vi "Script Editor Dialog.vi"(5 "VI Refnum":refnum<vi>, 7 "Name (\"\" to Use Uuid)":string="script_editor", 8 "Error In":errorcluster caption="Error in (no error)", 11 "Script":string="Data: Initialize\nInitialize Core Data\nEvents: Register\nUI: Initialize\nUI: Front Panel State >> Open\nstatus@a >> api@b -><register>") -> (0 "Error Out":errorcluster, 3 "Script Out":string)   [LabVIEW 2017]
uses:
  AdvanceAPI/CSM - Keywords.vi
  _Polymophic/CSM - Replace Marks in Messages.vi
  _Shared/Trim Single-line Text.vi
  Communicable State Machine.lvlib
  _ui/csm-ui-support.lvlib
panel:
  in  "Script List":i32(listbox)
  in  "Add Back":bool
  in  "Delete":bool
  in  "Add Front":bool
  in  "Replace":bool
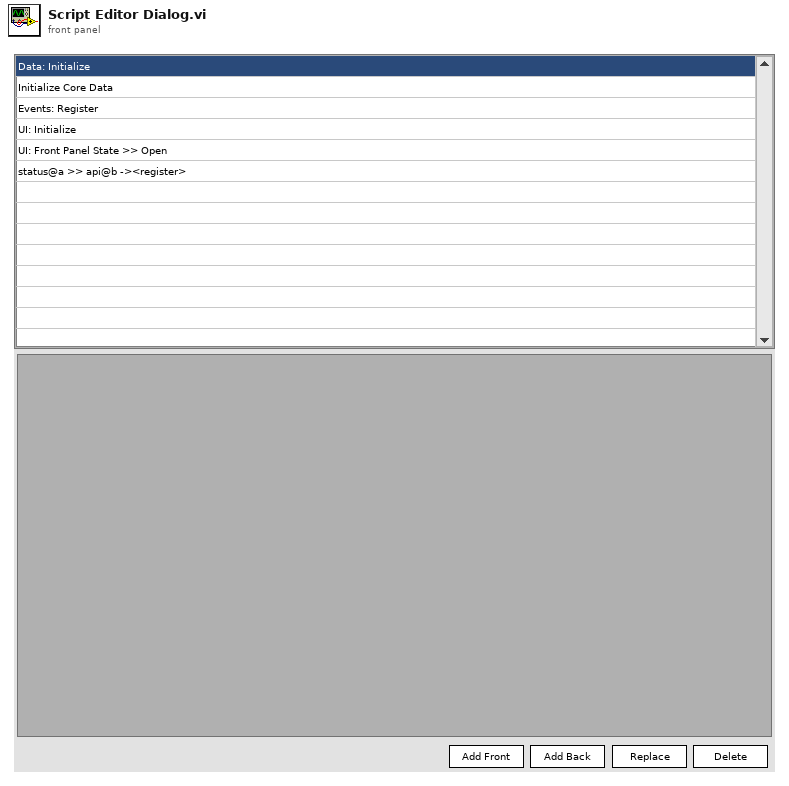
[diagram p1: front panel]
types:
  T1 = enum32{"Invalid", "Standard", "Closed", "Hidden", "Minimized", "Maximized"}
  T2 = enum32{"invalid app kind", "Development System", "Run Time System", "Student Edition", "Embedded LabVIEW", "Evaluation", "Custom"}
  T3 = typedef "Communicable State Machine.lvlib/_CSM_Response Source Message.ctl" = cluster{"‘State":string, "’Arguments":string, "’Error":errorcluster}
  T4 = cluster{"Current VI Reference":refnum<vi>, "Close Panel on Exit?":bool}
  T5 = cluster{"Core":cluster{"Current VI Reference":refnum<vi>, "Close Panel on Exit?":bool}, "Script":string}
  T6 = typedef "LVRectTypeDef.ctl" = cluster{"Left":i16, "Top":i16, "Right":i16, "Bottom":i16}
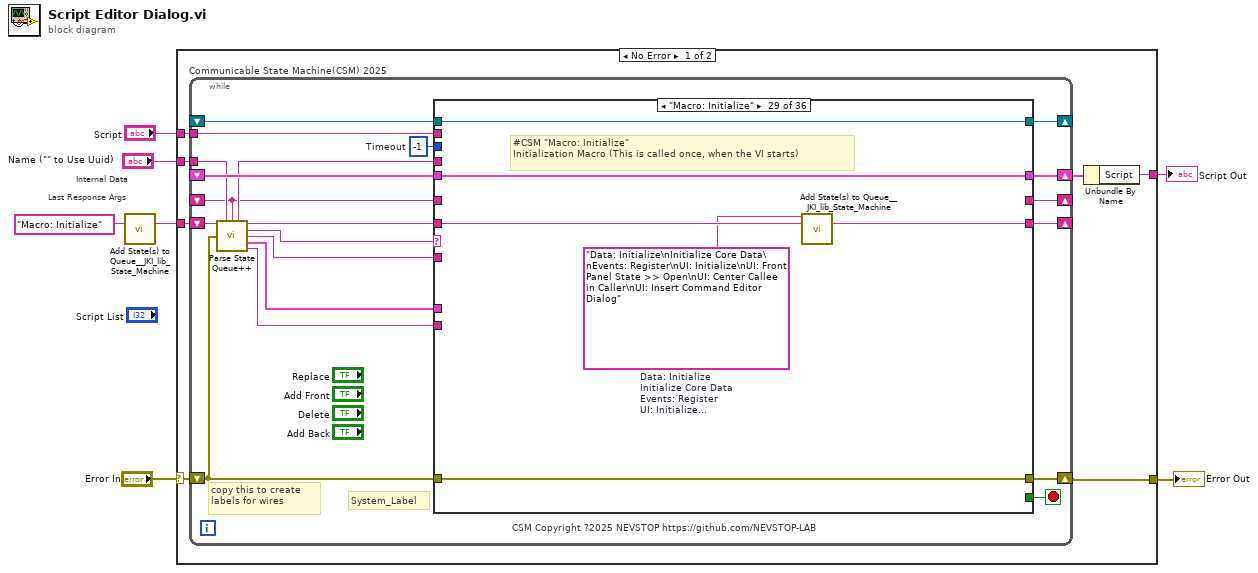
[diagram p0: block diagram]
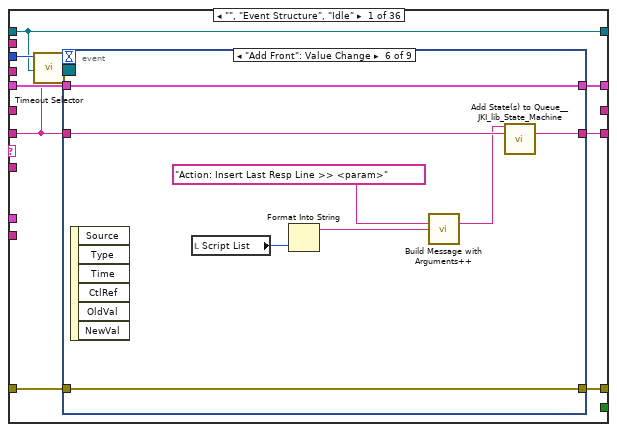
[diagram p2: hidden frame]
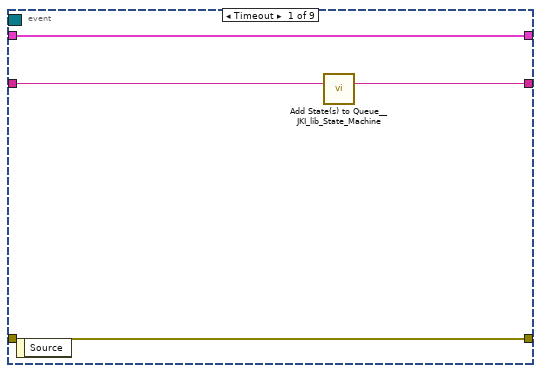
[diagram p3: hidden frame]
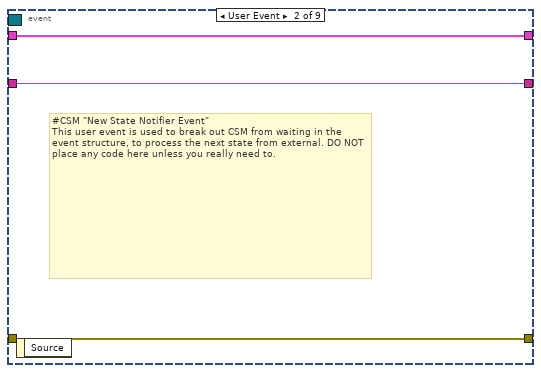
[diagram p4: hidden frame]
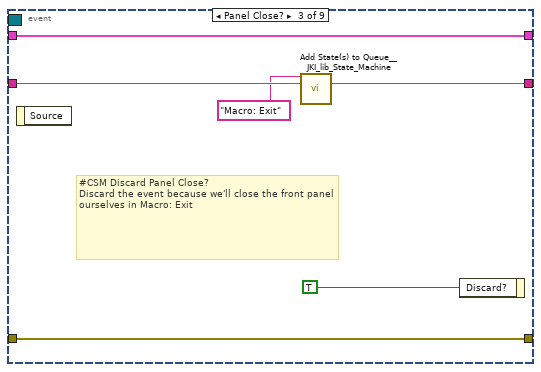
[diagram p5: hidden frame]
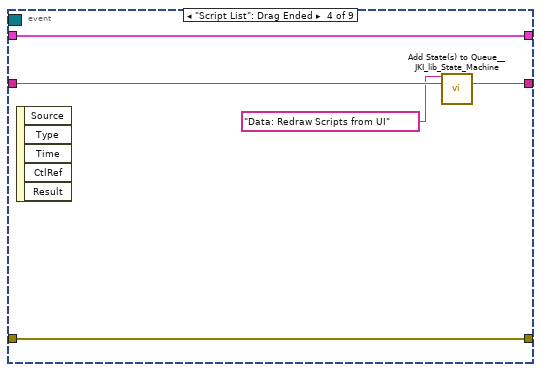
[diagram p6: hidden frame]
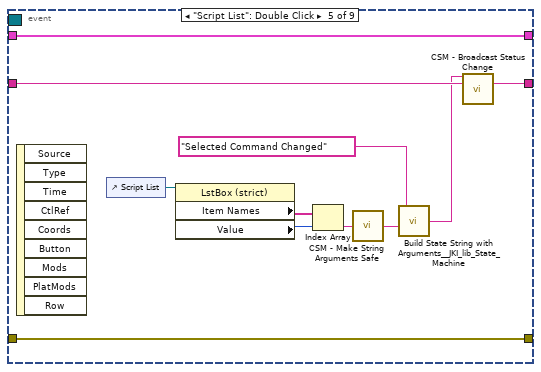
[diagram p7: hidden frame]
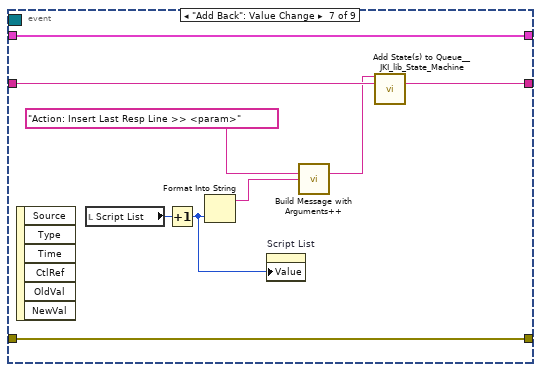
[diagram p8: hidden frame]
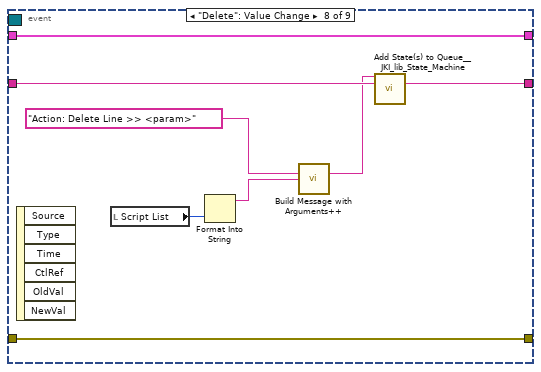
[diagram p9: hidden frame]
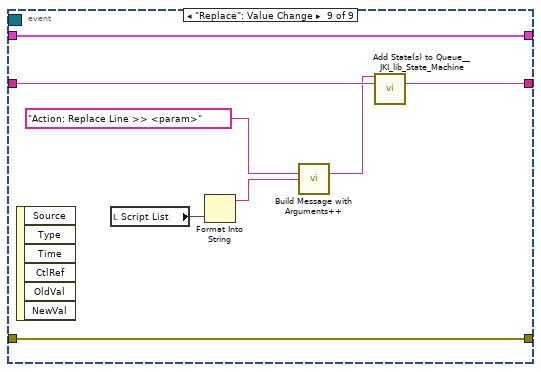
[diagram p10: hidden frame]
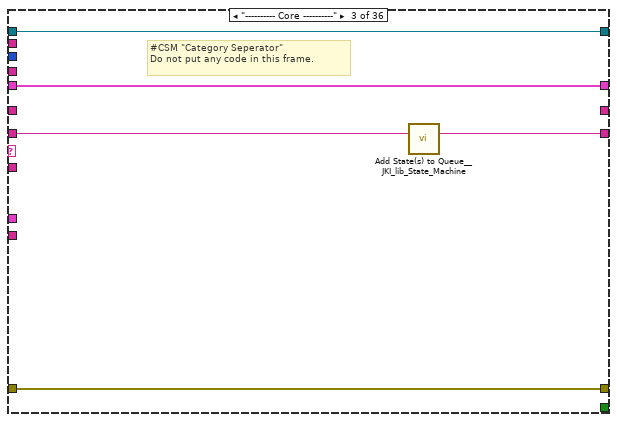
[diagram p12: hidden frame]
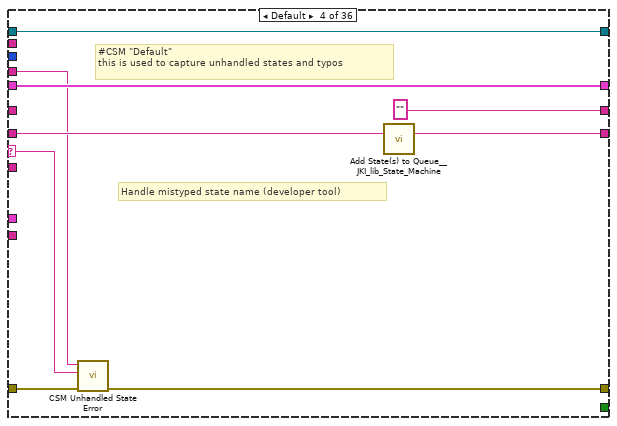
[diagram p13: hidden frame]
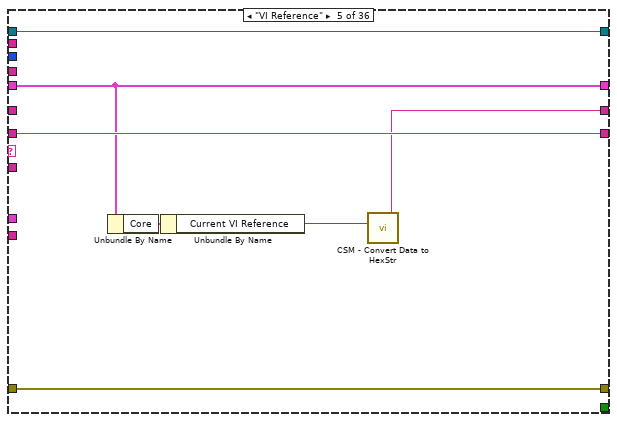
[diagram p14: hidden frame]
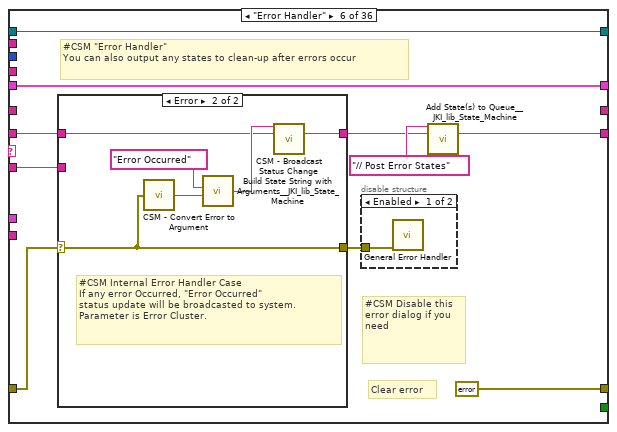
[diagram p15: hidden frame]
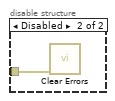
[diagram p16: hidden frame]
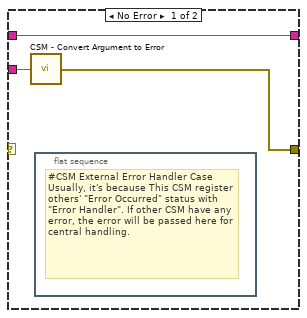
[diagram p17: hidden frame]
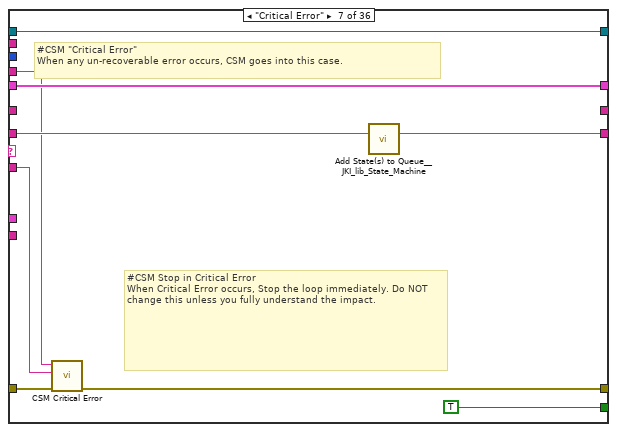
[diagram p18: hidden frame]
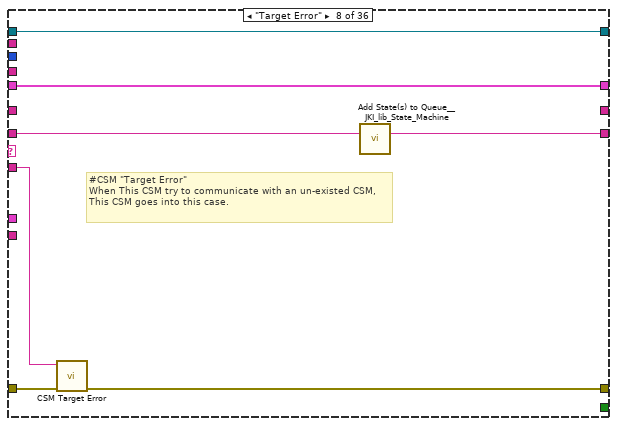
[diagram p19: hidden frame]
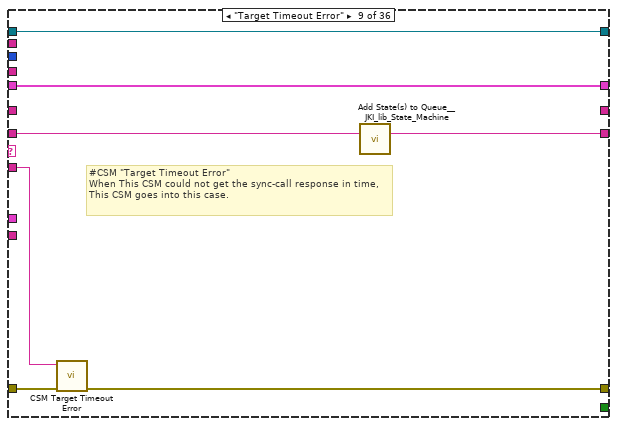
[diagram p20: hidden frame]
diagram:
  # "Last Response Args"
  # "Internal Data"
  n1 = call <vilib>:"Add State(s) to Queue__JKI_lib_State_Machine.vi"("State(s) in (\"\")"="Macro: Initialize" ("Init State(\"Macro: Initialize\")")) -> ("States Out"=w7:string)  [unwired: 14 in]
  n2 = case shown="No Error" "Error In" {
    selector: "Error In" -> [w11 w492]
    tunnel: w7 -> [w14 _]
    tunnel: "Name (\"\" to Use Uuid)" -> [w13 _]
    tunnel: [w12 w492] -> w4
    tunnel: [w9 w491] -> w2
    tunnel: "Script" -> [w8 w491]
    frame No Error {
      n3 = while "Communicable State Machine(CSM) 2025" {
        shift-right: [w29] -> w10
        shift-left: _ -> [w28]
        shift-right: [w32] -> w12
        shift-left: w11 -> [w26]
        shift-right: [w31] -> _
        shift-left: w14 -> [w33]
        tunnel: w13 -> [w22]
        shift-right: [w25] -> _
        shift-left: _ -> [w16]
        shift-right: [w24] -> _
        shift-left: _ -> [w23]
        tunnel: w8 -> [w15]
        stop <- w30 stop-if-true
        w27 = -1  # Timeout
        # "copy this to create labels for wires"
        # "System_Label"
        # "CSM Copyright ?2025 NEVSTOP https://github.com/NEVSTOP-LAB"
        n4 = call "Parse State Queue++.vi"("State Queue"=w33, "Name (\"\" to Use UUID)"=w22, "Response Arguments"=w16, "Previous Error"=w26) -> ("Name Used"=w17:string, "Remaining States"=w34:string, "Current State"=w21:string, "Arguments"=w20:string, "Additional Information"=w19:T3, "Source CSM"=w18:string)  [unwired: 6 in]
        n5 = case shown="\"Macro: Initialize\"" w21 {
          selector: w21 -> [_ _ _ w117 _ _ _ _ _ _ _ _ _ _ _ _ _ _ _ _ _ _ _ _ _ _ _ _ _ _ _ _ _ _ _ _]
          tunnel: w34 -> [w35 w108 w114 w122 w129 w135 w158 w164 w171 w180 w193 w208 w214 w219 w226 w233 w241 w246 w253 w257 w263 w270 w278 w281 w293 w309 w382 w404 w410 w424 w427 w430 w442 w460 w478 w490]
          tunnel: w20 -> [_ _ _ _ _ w134 w153 w163 w170 w179 _ _ _ _ _ _ _ _ _ _ _ _ _ _ w288 w303 _ _ _ _ _ w432 _ w456 w473 w485]
          tunnel: w28 -> [w42 w107 w111 w120 w128 w139 w159 w166 w173 w182 w192 w201 w212 w216 _ w232 w236 w243 w252 w256 w260 w266 w276 w285 w291 w305 w399 w401 w407 w421 w426 w436 w439 w458 w475 w487]
          tunnel: [w41 w109 w112 w115 w130 errorcluster {"status"=FALSE, "code"=0, "source"=""} ("error out") w154 w161 w168 w185 w194 w205 w211 w217 w223 w234 w237 w244 w247 w255 w261 w268 w279 w286 w289 w306 w381 w402 w408 w422 w428 w437 w440 w447 w476 w488] -> w32
          tunnel: w26 -> [w40 w109 w112 w123 w130 w136 w160 w162 w169 _ w194 w205 w211 w217 w223 w234 w238 w244 _ w258 w261 w268 w279 w286 w290 w307 _ w402 w408 w422 w428 w437 w440 _ w476 w488]
          tunnel: [w43 w108 w113 w121 w129 w131 w157 w167 w174 w181 w193 w207 w213 w218 w225 w233 w240 w245 w253 w257 w262 w269 w278 w282 w292 w308 w383 w403 w409 w423 w427 w431 w441 w459 w477 w489] -> w31
          tunnel: [_ _ _ _ _ _ TRUE _ _ _ _ _ TRUE _ _ _ _ _ _ _ _ _ _ _ _ _ _ _ _ _ _ _ _ _ _ _] -> w30
          tunnel: [w39 w107 w111 w120 w128 w139 w159 w166 w173 w183 w192 w206 w212 w216 w224 w228 w236 w243 w252 w256 w260 w266 w276 w285 w291 w305 w399 w401 w407 w421 w426 w434 w439 w458 w475 w487] -> w29
          tunnel: w27 -> [w38 _ _ _ _ _ _ _ _ _ _ _ _ _ _ _ _ _ _ _ _ _ _ _ _ _ _ _ _ _ _ _ _ _ _ _]
          tunnel: w18 -> [_ _ _ _ _ _ _ _ _ w177 _ _ _ _ _ _ _ _ _ _ _ _ _ _ _ _ _ _ _ _ _ _ _ _ _ _]
          tunnel: w19 -> [_ _ _ _ _ _ _ _ _ w184 _ _ _ _ _ _ _ _ _ _ _ _ _ _ _ _ _ _ _ _ _ _ _ _ _ _]
          tunnel: [_ _ _ "" w124 _ _ _ _ _ _ _ _ _ _ _ _ _ _ _ _ _ _ _ _ _ _ _ _ _ _ _ _ _ _ _] -> w25
          tunnel: [w37 w106 w110 w118 w127 w138 w155 w165 w172 w186 w191 w195 w209 w215 w221 w231 w235 w242 w251 w254 w259 w267 w277 w284 w287 w302 w398 w400 w405 w414 w425 w435 w438 w457 w474 w486] -> w24
          tunnel: w23 -> [w37 w106 w110 w118 w127 w138 w155 w165 w172 w186 w191 w195 w209 w215 w221 w231 w235 w242 _ w254 w259 w267 w277 w284 w287 w302 w398 w400 w405 w414 w425 w435 w438 w457 w474 w486]
          tunnel: w17 -> [_ _ _ w116 _ _ w152 _ _ _ _ _ _ _ _ _ _ _ w250 _ _ _ _ _ _ _ w387 _ _ w413 _ _ _ w446 w464 _]
          tunnel: w16 -> [_ _ _ _ _ _ _ _ _ _ _ _ _ _ _ _ _ _ _ _ _ _ _ _ _ _ _ _ _ _ _ _ _ _ _ _]
          tunnel: w15 -> [_ _ _ _ _ _ _ _ _ _ _ _ _ _ w220 _ _ _ _ _ _ _ _ _ _ _ _ _ _ _ _ _ _ _ _ _]
          frame "", "Event Structure", "Idle" {
            n6 = call "Timeout Selector.vi"("Remaining States"=w35, "Timeout Expected"=w38) -> ("Timeout"=w36:i32)  [unwired: 5 in]
            n7 = event shown="[5] \"Add Front\": Value Change" {
              selector: w37 -> [_ _ _ _ _ _ _ _ _]
              dyn-events: _ -> [_ _ _ _ _ _ _ _ _]
              timeout: w36 -> [_ _ _ _ _ _ _ _ _]
              tunnel: w35 -> [w47 w49 w56 w58 w69 w77 w86 w94 w102]
              tunnel: [w46 w49 w55 w59 w70 w78 w87 w95 w103] -> w43
              tunnel: w42 -> [w44 w50 w53 w60 w71 w79 w88 w96 w104]
              tunnel: [w45 w48 w54 w61 w72 w80 w89 w97 w105] -> w41
              tunnel: w40 -> [w45 w48 w54 w61 w72 w80 w89 w97 w105]
              tunnel: [w44 w50 w53 w60 w71 w79 w88 w96 w104] -> w39
              event Timeout {
                n8 = event-data() -> ()  [unwired: 1 in, 1 out]
                n9 = call <vilib>:"Add State(s) to Queue__JKI_lib_State_Machine.vi"("State(s) in (\"\")"=w47) -> ("States Out"=w46:string)  [unwired: 14 in]
              }
              event User Event {
                # "#CSM \"New State Notifier Event\"\nThis user event is used to break out CSM from waiting in the event structure, to process the next state from external. DO NOT place any code here unless you really need to."
                n10 = event-data() -> ()  [unwired: 1 in, 1 out]
              }
              event Panel Close? {
                # "#CSM Discard Panel Close?\nDiscard the event because we'll close the front panel ourselves in Macro: Exit"
                n11 = event-data() -> ()  [unwired: 1 in, 1 out]
                n12 = call <vilib>:"Add State(s) to Queue__JKI_lib_State_Machine.vi"("State(s) in Front (\"\")"="Macro: Exit", "State(s) in (\"\")"=w56) -> ("States Out"=w55:string)  [unwired: 13 in]
                n13 = event-data("Discard?"=TRUE) -> ()  [unwired: 1 in, 1 out]
              }
              event "Script List": Drag Ended {
                n14 = event-data() -> ()  [unwired: 1 in, 5 out]
                n15 = call <vilib>:"Add State(s) to Queue__JKI_lib_State_Machine.vi"("State(s) in Front (\"\")"="Data: Redraw Scripts from UI" ("State(s) in Front (\"\")"), "State(s) in (\"\")"=w58) -> ("States Out"=w59:string)  [unwired: 13 in]
              }
              event "Script List": Double Click {
                n16 = event-data() -> ()  [unwired: 1 in, 9 out]
                n17 = control-ref of="Script List"() -> (w65:refnum<vi>)
                n18 = property class="LstBox (strict)"(reference=w65) -> ("Item Names"=w68:string[], "Value"=w67:i32)  [unwired: 1 in, 2 out]
                n19 = Index Array(array=w68, index=w67) -> (element=w66:string)
                n20 = call "CSM - Make String Arguments Safe.vi"("Argument String"=w66) -> ("Safe Argument String"=w64:string)  [unwired: 8 in]
                n21 = call <vilib>:"Build State String with Arguments__JKI_lib_State_Machine.vi"("Arguments (\"\")"=w64, "State"="Selected Command Changed") -> ("State with Arguments"=w62:string)  [unwired: 4 in]
                n22 = call "CSM - Broadcast Status Change.vi"("Status With Arguments"=w62, "State Queue"=w69) -> ("Remaining States"=w70:string)  [unwired: 13 in]
              }
              event "Add Front": Value Change {
                n23 = event-data() -> ()  [unwired: 1 in, 6 out]
                n24 = local read "Script List"() -> (w74:i32)
                n25 = Format Into String(w74) -> (resulting string=w73:string)  [unwired: 3 in, 1 out]
                n26 = call-poly "Build Message with Arguments++.vi"("States With Replace Token"="Action: Insert Last Resp Line >> <param>" ("State(s) in Front (\"\")"), "<param>"=w73) -> ("States"=w75:string)  [unwired: 13 in]
                n27 = call <vilib>:"Add State(s) to Queue__JKI_lib_State_Machine.vi"("State(s) in Front (\"\")"=w75, "State(s) in (\"\")"=w77) -> ("States Out"=w78:string)  [unwired: 13 in]
              }
              event "Add Back": Value Change {
                n28 = event-data() -> ()  [unwired: 1 in, 6 out]
                n29 = local read "Script List"() -> (w83:i32)
                n30 = Increment(x=w83) -> (x+1=w81:i32)
                n31 = Format Into String(w81) -> (resulting string=w82:string)  [unwired: 3 in, 1 out]
                n32 = property on="Script List" class="LstBox (strict)"("Value"=w81) -> ()  [unwired: 2 in, 2 out]
                n33 = call-poly "Build Message with Arguments++.vi"("States With Replace Token"="Action: Insert Last Resp Line >> <param>" ("State(s) in Front (\"\")"), "<param>"=w82) -> ("States"=w84:string)  [unwired: 13 in]
                n34 = call <vilib>:"Add State(s) to Queue__JKI_lib_State_Machine.vi"("State(s) in Front (\"\")"=w84, "State(s) in (\"\")"=w86) -> ("States Out"=w87:string)  [unwired: 13 in]
              }
              event "Delete": Value Change {
                n35 = event-data() -> ()  [unwired: 1 in, 6 out]
                n36 = local read "Script List"() -> (w91:i32)
                n37 = Format Into String(w91) -> (resulting string=w90:string)  [unwired: 3 in, 1 out]
                n38 = call-poly "Build Message with Arguments++.vi"("States With Replace Token"="Action: Delete Line >> <param>" ("State(s) in Front (\"\")"), "<param>"=w90) -> ("States"=w92:string)  [unwired: 13 in]
                n39 = call <vilib>:"Add State(s) to Queue__JKI_lib_State_Machine.vi"("State(s) in Front (\"\")"=w92, "State(s) in (\"\")"=w94) -> ("States Out"=w95:string)  [unwired: 13 in]
              }
              event "Replace": Value Change {
                n40 = event-data() -> ()  [unwired: 1 in, 6 out]
                n41 = local read "Script List"() -> (w99:i32)
                n42 = Format Into String(w99) -> (resulting string=w98:string)  [unwired: 3 in, 1 out]
                n43 = call-poly "Build Message with Arguments++.vi"("States With Replace Token"="Action: Replace Line >> <param>" ("State(s) in Front (\"\")"), "<param>"=w98) -> ("States"=w100:string)  [unwired: 13 in]
                n44 = call <vilib>:"Add State(s) to Queue__JKI_lib_State_Machine.vi"("State(s) in Front (\"\")"=w100, "State(s) in (\"\")"=w102) -> ("States Out"=w103:string)  [unwired: 13 in]
              }
            }
          }
          frame "CSM Documentation" {
            # "#CSM README FIRST\n\nCommunicable State Machine(CSM) is a LabVIEW application framework that builds upon JKI State Machine(JKISM). It follows the pattern of JKISM and extends the keywords to describe message communication between modules, including concepts such as Sync-Message, Async-Message, Subscription/Unsubscription of status - essential elements for creating reusable code modules. For more information, please visit the CSM wiki: https://nevstop-lab.github.io/CSM-Wiki/\n\nFor instructions on JKI State Machine, visit: http://jki.net/state-machine/\nFor information about CSM, visit: https://github.com/NEVSTOP-LAB"
            # "#CSM \"Documentation\"\nCase for holding CSM Documenation"
          }
          frame "---------- Core ----------" {
            # "#CSM \"Category Seperator\"\nDo not put any code in this frame."
            n45 = call <vilib>:"Add State(s) to Queue__JKI_lib_State_Machine.vi"("State(s) in (\"\")"=w114) -> ("States Out"=w113:string)  [unwired: 14 in]
          }
          frame Default {
            # "#CSM \"Default\"\nthis is used to capture unhandled states and typos"
            # "Handle mistyped state name (developer tool)"
            n46 = call "CSM Unhandled State Error.vi"("error in (no error)"=w123, "Undefined State"=w117, "CSM Name"=w116) -> ("error out"=w115:errorcluster)  [unwired: 8 in]
            n47 = call <vilib>:"Add State(s) to Queue__JKI_lib_State_Machine.vi"("State(s) in (\"\")"=w122) -> ("States Out"=w121:string)  [unwired: 14 in]
          }
          frame "VI Reference" {
            n48 = Unbundle By Name(w128) -> ("Core"=w126:T4)
            n49 = Unbundle By Name(w126) -> ("Current VI Reference"=w125:refnum<vi>)
            n50 = call "CSM - Convert Data to HexStr.vi"("Variant"=w125) -> ("HEX String (0-9,A-F)"=w124:string)  [unwired: 8 in]
          }
          frame "Error Handler" {
            # "#CSM Disable this error dialog if you need"
            # "#CSM \"Error Handler\"\nYou can also output any states to clean-up after errors occur"
            # "Clear error"
            n51 = case shown="Error" w136 {
              selector: w136 -> [_ w146]
              tunnel: [w145 w148] -> w132
              tunnel: w135 -> [w145 w147]
              tunnel: w134 -> [w144 _]
              tunnel: [w143 w146] -> w137
              frame No Error {
                n52 = call "CSM - Convert Argument to Error.vi"("Argument"=w144) -> ("Error"=w143:errorcluster)  [unwired: 4 in]
                n53 = flat-sequence {
                  frame #0 {
                    # "#CSM External Error Handler Case\nUsually, it's because This CSM register others' \"Error Occurred\" status with \"Error Handler\". If other CSM have any error, the error will be passed here for central handling."
                  }
                }
              }
              frame Error {
                # "#CSM Internal Error Handler Case \nIf any error Occurred, \"Error Occurred\" \nstatus update will be broadcasted to system.\nParameter is Error Cluster."
                n54 = call "CSM - Convert Error to Argument.vi"("Error"=w146) -> ("Argument"=w150:string)  [unwired: 4 in]
                n55 = call <vilib>:"Build State String with Arguments__JKI_lib_State_Machine.vi"("Arguments (\"\")"=w150, "State"="Error Occurred" ("Status with Arguments")) -> ("State with Arguments"=w149:string)  [unwired: 4 in]
                n56 = call "CSM - Broadcast Status Change.vi"("Status With Arguments"=w149, "State Queue"=w147) -> ("Remaining States"=w148:string)  [unwired: 13 in]
              }
            }
            n57 = disable-structure shown="Enabled" {
              disable-tunnel: w137 -> [w141 w142]
              frame Enabled {
                n58 = call <vilib>:"General Error Handler.vi"("error in (no error)"=w141) -> ()  [unwired: 10 in, 5 out]
              }
              frame Disabled {
                n59 = call <vilib>:"Clear Errors.vi"("error in (no error)"=w142) -> ()  [unwired: 5 in, 2 out]
              }
            }
            n60 = call <vilib>:"Add State(s) to Queue__JKI_lib_State_Machine.vi"("State(s) in Front (\"\")"="// Post Error States", "State(s) in (\"\")"=w132) -> ("States Out"=w131:string)  [unwired: 13 in]
          }
          frame "Critical Error" {
            # "#CSM Stop in Critical Error\nWhen Critical Error occurs, Stop the loop immediately. Do NOT change this unless you fully understand the impact."
            # "#CSM \"Critical Error\"\nWhen any un-recoverable error occurs, CSM goes into this case."
            n61 = call "CSM Critical Error.vi"("error in (no error)"=w160, "Arugments (As Reason)"=w153, "CSM Name"=w152) -> ("error out"=w154:errorcluster)  [unwired: 8 in]
            n62 = call <vilib>:"Add State(s) to Queue__JKI_lib_State_Machine.vi"("State(s) in (\"\")"=w158) -> ("States Out"=w157:string)  [unwired: 14 in]
          }
          frame "Target Error" {
            # "#CSM \"Target Error\"\nWhen This CSM try to communicate with an un-existed CSM, This CSM goes into this case."
            n63 = call "CSM Target Error.vi"("error in (no error)"=w162, "Arguments (As CSM Name)"=w163) -> ("error out"=w161:errorcluster)  [unwired: 9 in]
            n64 = call <vilib>:"Add State(s) to Queue__JKI_lib_State_Machine.vi"("State(s) in (\"\")"=w164) -> ("States Out"=w167:string)  [unwired: 14 in]
          }
          frame "Target Timeout Error" {
            # "#CSM \"Target Timeout Error\"\nWhen This CSM could not get the sync-call response in time, This CSM goes into this case."
            n65 = call "CSM Target Timeout Error.vi"("error in (no error)"=w169, "Arguments (As CSM Name)"=w170) -> ("error out"=w168:errorcluster)  [unwired: 9 in]
            n66 = call <vilib>:"Add State(s) to Queue__JKI_lib_State_Machine.vi"("State(s) in (\"\")"=w171) -> ("States Out"=w174:string)  [unwired: 14 in]
          }
          frame "Async Response", "Response" {
            n67 = Unbundle(w184) -> ("‘State"=w178:string, "’Arguments"=w176:string, "’Error"=w175:errorcluster)
            n68 = case shown="Default" w178 {
              tunnel: [w190] -> w185
              tunnel: w175 -> [w190]
              tunnel: [w189] -> w183
              tunnel: w182 -> [w189]
              tunnel: [w187] -> w181
              tunnel: w180 -> [w188]
              tunnel: w179 -> [_]
              tunnel: w177 -> [_]
              tunnel: w176 -> [_]
              frame Default {
                # "#CSM Response Comments\nAfter Message is executed, CSM goes to this state for receive the response.\n    For Async Message(->), \"Async Response\" is used. This CSM will goes to \"Async Message Posted\" immediately and receive the \"Async Response\" after the callee finishes the message.\n    For Sync Message(@),  This CSM will wait until the message is done and immediately goes to \"Response\""
                # "#CSM \"Async Response\"\nHandle Async-call Response (\"Async Response\" for ->)"
                # "#CSM \"Response\"\nHandle Sync-call Response (\"Response\" for -@)"
                n69 = call <vilib>:"Add State(s) to Queue__JKI_lib_State_Machine.vi"("State(s) in (\"\")"=w188) -> ("States Out"=w187:string)  [unwired: 14 in]
              }
            }
          }
          frame "Async Message Posted" {
            # "#CSM \"Async Message Posted\"\nAfter Async Message is posted (-> or ->| ), CSM goes to this state for post-action.\nYou can use Argument - State to tell which Async Message is called."
          }
          frame "Initialize Core Data" {
            # "#CSM \"Initialize Core Data\"\nThis is used to determine panel behavior on exit"
            # "originally closed?"
            # "exe?"
            # "If panel starts closed or is an EXE, then close it when we exit"
            n70 = property class="VI"() -> ("FP.State"=w198:T1)  [unwired: 2 in, 2 out]
            n71 = property class="App"() -> ("App.Kind"=w204:T2)  [unwired: 2 in, 2 out]
            n72 = control-ref of="Current VI Reference"() -> (w199:refnum<vi>)
            n73 = Equal?(x=w198, y=T1."Closed" ("Front Panel Window:State")) -> (x = y?=w196:bool)
            n74 = Equal?(x=w204, y=T2."Run Time System" ("Application:Kind")) -> (x = y?=w202:bool)
            n75 = Or(x=w196, y=w202) -> (x .or. y?=w200:bool)
            n76 = Bundle By Name(cluster=w201, "Core.Current VI Reference"=w199, "Core.Close Panel on Exit?"=w200) -> (w206:T5)
            n77 = call <vilib>:"Add State(s) to Queue__JKI_lib_State_Machine.vi"("State(s) in (\"\")"=w208) -> ("States Out"=w207:string)  [unwired: 14 in]
          }
          frame "Exit" {
            # "#CSM \"Exit\"\nCase for exiting the loop. No errors that occur here will be handled."
            n78 = call <vilib>:"Add State(s) to Queue__JKI_lib_State_Machine.vi"("State(s) in (\"\")"=w214) -> ("States Out"=w213:string)  [unwired: 14 in]
          }
          frame "---------- Data ----------" {
            # "#CSM \"Category Seperator\"\nDo not put any code in this frame."
            n79 = call <vilib>:"Add State(s) to Queue__JKI_lib_State_Machine.vi"("State(s) in (\"\")"=w219) -> ("States Out"=w218:string)  [unwired: 14 in]
          }
          frame "Data: Initialize" {
            w222 = T4 {"Current VI Reference"=refnum, "Close Panel on Exit?"=FALSE}  # Core
            n80 = Bundle("Core"=w222, "Script"=w220) -> (w224:T5)  [unwired: 1 in]
            n81 = call <vilib>:"Add State(s) to Queue__JKI_lib_State_Machine.vi"("State(s) in (\"\")"=w226) -> ("States Out"=w225:string)  [unwired: 14 in]
          }
          frame "Data: Redraw Scripts from UI" {
            n82 = control-ref of="Script List"() -> (w230:refnum<vi>)
            n83 = property class="LstBox (strict)"(reference=w230) -> ("Item Names"=w229:string[])  [unwired: 1 in, 2 out]
            n84 = call "CSM - Compact Multiple States.vi"("Multiple States"=w229) -> ("States"=w227:string)  [unwired: 9 in]
            n85 = Bundle By Name(cluster=w232, "Script"=w227) -> (w228:T5)
          }
          frame "Data: Cleanup" {
            # "Cleanup any data and references, here.\n(this is called automatically, by the Macro: Exit)"
            n86 = Unbundle By Name(w236) -> ("Core.Current VI Reference"=w239:refnum<vi>)
            n87 = Close Reference(reference=w239, error in (no error)=w238) -> (error out=w237:errorcluster)
            n88 = call <vilib>:"Add State(s) to Queue__JKI_lib_State_Machine.vi"("State(s) in (\"\")"=w241) -> ("States Out"=w240:string)  [unwired: 14 in]
          }
          frame "---------- Events ----------" {
            # "#CSM \"Category Seperator\"\nDo not put any code in this frame."
            n89 = call <vilib>:"Add State(s) to Queue__JKI_lib_State_Machine.vi"("State(s) in (\"\")"=w246) -> ("States Out"=w245:string)  [unwired: 14 in]
          }
          frame "Events: Register" {
            # "#CSM \"Events: Register\"\nRegister user event. New Message Event is registered to break CSM waiting in event structure by default."
            # "#CSM Register New Message Event\nRegister message event to break Waiting in Event structure."
            n90 = call "CSM - Get New State Notifier Event.vi"("Name (\"\" to Use UUID)"=w250) -> ("error out"=w248:errorcluster, "New State Notifier Event"=w249:refnum<user-event>)  [unwired: 9 in]
            n91 = register-events(error in=w248, w249) -> (reference out=w251:refnum<event-registration>, error out=w247:errorcluster)  [unwired: 1 in]
          }
          frame "Events: Unregister" {
            # "#CSM \"Events: Unregister\"\nUnregister user event."
            n92 = Unregister For Events(event registration refnum=w254, error in=w258) -> (error out=w255:errorcluster)
          }
          frame "---------- UI ----------" {
            # "#CSM \"Category Seperator\"\nDo not put any code in this frame."
            n93 = call <vilib>:"Add State(s) to Queue__JKI_lib_State_Machine.vi"("State(s) in (\"\")"=w263) -> ("States Out"=w262:string)  [unwired: 14 in]
          }
          frame "UI: Initialize" {
            # "#CSM \"UI: Initialize\"\nInitialize the User Interface, here.\n(this is called automatically, by the Macro: Init)"
            n94 = Unbundle By Name(w266) -> ("Script"=w265:string)
            n95 = call "CSM - Break Down Multiple States String.vi"("States"=w265) -> ("Multiple States"=w264:string[])  [unwired: 10 in]
            n96 = property on="Script List" class="LstBox (strict)"("Item Names"=w264) -> ()  [unwired: 2 in, 2 out]
            n97 = call <vilib>:"Add State(s) to Queue__JKI_lib_State_Machine.vi"("State(s) in (\"\")"=w270) -> ("States Out"=w269:string)  [unwired: 14 in]
          }
          frame "UI: Center Callee in Caller" {
            n98 = Unbundle By Name(w276) -> ("Core.Current VI Reference"=w273:refnum<vi>)
            n99 = property class="VI"(reference="VI Refnum") -> (error out=w271:errorcluster, "BDWin.Bounds"=w272:T6)  [unwired: 1 in, 1 out]
            n100 = call "Center Callee in Window Bounds.vi"("Callee VI Refnum (Caller)"=w273, "Block Diagram Window:Window Bounds"=w272) -> ("Error Out"=w275:errorcluster)  [unwired: 9 in]
            n101 = call <vilib>:"Clear Errors.vi"("error in (no error)"=w271) -> ()  [unwired: 5 in, 2 out]
            n102 = call <vilib>:"Clear Errors.vi"("error in (no error)"=w275) -> ()  [unwired: 5 in, 2 out]
          }
          frame "UI: Refresh Inputs" {
            n103 = call <vilib>:"Build State String with Arguments__JKI_lib_State_Machine.vi"("State"="") -> ("State with Arguments"=w280:string)  [unwired: 5 in]
            n104 = call <vilib>:"Add State(s) to Queue__JKI_lib_State_Machine.vi"("State(s) in Front (\"\")"=w280, "State(s) in (\"\")"=w281) -> ("States Out"=w282:string)  [unwired: 13 in]
          }
          frame "UI: Cursor Set" {
            # "#CSM \"UI: Cursor Set\"\nSet and Unset Cursor Busy.\n(Usage: \"UI: Cursor Set >> Busy|Idle\")"
            # "Argument"
            n105 = disable-structure shown="Default" {
              disable-tunnel: w290 -> [w296 w301]
              disable-tunnel: [w295 w301] -> w289
              disable-tunnel: w288 -> [w294 _]
              frame condition #0 (active) {
                n106 = case shown="\"Idle\", Default" w294 {
                  tunnel: w296 -> [w298 w300]
                  tunnel: [w297 w299] -> w295
                  frame "Idle", Default {
                    n107 = call <vilib>:"Unset Busy.vi"("error in (no error)"=w298) -> ("error out"=w297:errorcluster)  [unwired: 10 in]
                  }
                  frame "Busy" {
                    n108 = call <vilib>:"Set Busy.vi"("error in (no error)"=w300) -> ("error out"=w299:errorcluster)  [unwired: 9 in, 1 out]
                  }
                }
              }
              frame condition #1 {
              }
            }
            n109 = call <vilib>:"Add State(s) to Queue__JKI_lib_State_Machine.vi"("State(s) in (\"\")"=w293) -> ("States Out"=w292:string)  [unwired: 14 in]
          }
          frame "UI: Front Panel State" {
            # "#CSM \"UI: Front Panel State\"\nSet Front Panel Open or Closed\n(Usage: \"UI: Front Panel State >> Open|Close\")"
            # "Argument"
            n110 = Unbundle By Name(w305) -> ("Core.Current VI Reference"=w304:refnum<vi>)
            n111 = call <vilib>:"Add State(s) to Queue__JKI_lib_State_Machine.vi"("State(s) in (\"\")"=w309) -> ("States Out"=w308:string)  [unwired: 14 in]
            n112 = case shown="\"Close\", \"Closed\"" w303 {
              tunnel: w307 -> [w315 w330 w341 w354 w367]
              tunnel: [w317 w331 w343 w356 w369] -> w306
              tunnel: w304 -> [w316 w328 w342 w355 w368]
              frame "Open", "Standard", Default {
                w310 = T1."Standard" ("State")
                n113 = property class="VI"(reference=w316, error in=w315) -> (reference out=w313:refnum<vi>, error out=w314:errorcluster, "FP.State"=w312:T1)
                n114 = Not Equal?(x=w312, y=w310) -> (x != y?=w311:bool)
                n115 = case shown="True" w311 {
                  tunnel: [w321 w323] -> w317
                  tunnel: w314 -> [w320 w323]
                  tunnel: w313 -> [w319 _]
                  tunnel: w310 -> [w318 _]
                  frame True {
                    n116 = invoke class="VI" method="FP.Open"(reference=w319, error in=w320, "Activate"=TRUE, "State"=w318) -> (error out=w321:errorcluster)  [unwired: 1 in, 4 out]
                  }
                  frame False {
                  }
                }
              }
              frame "Close", "Closed" {
                n117 = property class="VI"(reference=w328, error in=w330) -> (reference out=w327:refnum<vi>, error out=w329:errorcluster, "FP.State"=w325:T1)
                n118 = Not Equal?(x=w325, y=T1."Closed" ("Front Panel Window:State")) -> (x != y?=w324:bool)
                n119 = case shown="False" w324 {
                  tunnel: [w332 w335] -> w331
                  tunnel: w329 -> [w332 w334]
                  tunnel: w327 -> [_ w333]
                  frame False {
                  }
                  frame True {
                    n120 = invoke class="VI" method="FP.Close"(reference=w333, error in=w334) -> (error out=w335:errorcluster)  [unwired: 1 in, 2 out]
                  }
                }
              }
              frame "Hidden", "Hide" {
                w336 = T1."Hidden" ("State")
                n121 = property class="VI"(reference=w342, error in=w341) -> (reference out=w339:refnum<vi>, error out=w340:errorcluster, "FP.State"=w338:T1)
                n122 = Not Equal?(x=w338, y=w336) -> (x != y?=w337:bool)
                n123 = case shown="True" w337 {
                  tunnel: [w347 w348] -> w343
                  tunnel: w340 -> [w346 w348]
                  tunnel: w339 -> [w345 _]
                  tunnel: w336 -> [w344 _]
                  frame True {
                    n124 = invoke class="VI" method="FP.Open"(reference=w345, error in=w346, "State"=w344) -> (error out=w347:errorcluster)  [unwired: 2 in, 4 out]
                  }
                  frame False {
                  }
                }
              }
              frame "Minimize", "Minimized" {
                w349 = T1."Minimized" ("State")
                n125 = property class="VI"(reference=w355, error in=w354) -> (reference out=w352:refnum<vi>, error out=w353:errorcluster, "FP.State"=w351:T1)
                n126 = Not Equal?(x=w351, y=w349) -> (x != y?=w350:bool)
                n127 = case shown="True" w350 {
                  tunnel: [w360 w361] -> w356
                  tunnel: w353 -> [w359 w361]
                  tunnel: w352 -> [w358 _]
                  tunnel: w349 -> [w357 _]
                  frame True {
                    n128 = invoke class="VI" method="FP.Open"(reference=w358, error in=w359, "State"=w357) -> (error out=w360:errorcluster)  [unwired: 2 in, 4 out]
                  }
                  frame False {
                  }
                }
              }
              frame "Maximize", "Maximized" {
                w362 = T1."Maximized" ("State")
                n129 = property class="VI"(reference=w368, error in=w367) -> (reference out=w365:refnum<vi>, error out=w366:errorcluster, "FP.State"=w364:T1)
                n130 = Not Equal?(x=w364, y=w362) -> (x != y?=w363:bool)
                n131 = case shown="True" w363 {
                  tunnel: [w373 w374] -> w369
                  tunnel: w366 -> [w372 w374]
                  tunnel: w365 -> [w371 _]
                  tunnel: w362 -> [w370 _]
                  frame True {
                    n132 = invoke class="VI" method="FP.Open"(reference=w371, error in=w372, "State"=w370) -> (error out=w373:errorcluster)  [unwired: 2 in, 4 out]
                  }
                  frame False {
                  }
                }
              }
            }
          }
          frame "UI: Insert Command Editor Dialog" {
            n133 = vi-ref "Command Editor Dialog.vi"() -> (w388:refnum<vi>)
            n134 = property class="VI (strict)"(reference=w388) -> (reference out=w393:refnum<vi>, error out=w391:errorcluster, "Path"=w390:path)  [unwired: 1 in]
            n135 = Open VI Reference(type specifier VI Refnum (for type only)=w393, vi path=w390, options=128, error in (no error)=w391) -> (vi reference=w392:refnum<vi>, error out=w389:errorcluster)  [unwired: 2 in]
            n136 = call "Concatenate Submodule Name.vi"("Module Name"="CmdEditor", "Group Name"=w387) -> ("Submodule Name"=w375:string)  [unwired: 9 in]
            n137 = call-by-ref "Start Asynchronous Call"(reference=w392, error in=w389, "Name(\"\" to use uuid)"=w375, "CSM States"="" ("Command")) -> (reference out=w396:refnum<vi>, error out=w395:errorcluster)  [unwired: 8 in, 2 out]
            n138 = Close Reference(reference=w396, error in (no error)=w395) -> (error out=w386:errorcluster)
            n139 = call "CSM - Wait for Module to Be Alive.vi"("CSM Name"=w375, "error in (no error)"=w386) -> ("CSM Name (Dup)"=w384:string, "error out"=w385:errorcluster)  [unwired: 11 in, 1 out]
            n140 = call "CSM - Module VI Reference.vi"("error in (no error)"=w385, "CSM Name"=w384) -> ("error out"=w376:errorcluster, "CSM Module VIRef"=w379:refnum<vi>)  [unwired: 8 in]
            n141 = invoke on="Sub Panel" class="SubPnl" method="Insert VI"(error in=w376, "VI Ref"=w379) -> (error out=w381:errorcluster)  [unwired: 2 in, 3 out]
            n142 = call-poly "Build Message with Arguments++.vi"("States With Replace Token"="Selected Command changed@* >> API: Set Command@<target>-><register>" ("State(s) in Front (\"\")"), "<target>"=w375) -> ("States"=w378:string)  [unwired: 13 in]
            n143 = call <vilib>:"Add State(s) to Queue__JKI_lib_State_Machine.vi"("State(s) in Front (\"\")"=w378, "State(s) in (\"\")"=w382) -> ("States Out"=w383:string)  [unwired: 13 in]
          }
          frame "---------- Macro ----------" {
            # "#CSM \"Category Seperator\"\nDo not put any code in this frame."
            n144 = call <vilib>:"Add State(s) to Queue__JKI_lib_State_Machine.vi"("State(s) in (\"\")"=w404) -> ("States Out"=w403:string)  [unwired: 14 in]
          }
          frame "Macro: Initialize" {
            w406 = "Data: Initialize\nInitialize Core Data\nEvents: Register\nUI: Initialize\nUI: Front Panel State >> Open\nUI: Center Callee in Caller\nUI: Insert Command Editor Dialog"  # Data: Initialize Initialize Core Data Events: Register UI: Initialize UI: Front Panel State >> Open UI: Center Callee in Caller UI: Insert Command Editor Dialog
            # "#CSM \"Macro: Initialize\"\nInitialization Macro (This is called once, when the VI starts)"
            n145 = call <vilib>:"Add State(s) to Queue__JKI_lib_State_Machine.vi"("State(s) in Front (\"\")"=w406, "State(s) in (\"\")"=w410) -> ("States Out"=w409:string)  [unwired: 13 in]
          }
          frame "Macro: Exit" {
            # "#CSM \"Macro: Exit\"\nExit Macro (This is called once, when the VI exits)"
            n146 = Unbundle By Name(w421) -> ("Core.Close Panel on Exit?"=w420:bool)
            n147 = call "CSM - List Submodules.vi"("Parent Name"=w413) -> ("Submodules"=w412:string[])  [unwired: 8 in, 2 out]
            n148 = call "CSM - Build Exit Messages of CSMs.vi"("CSMs"=w412) -> ("States"=w411:string)  [unwired: 14 in]
            n149 = Select(t="UI: Front Panel State >> Close", s=w420, f="") -> (s? t:f=w417:string)
            n150 = call <vilib>:"Add State(s) to Queue__JKI_lib_State_Machine.vi"("State(s) in Front (\"\")"=w411, "State(s) in (\"\")"=w417, "State(s) at Back (\"\")"="Data: Cleanup\nEvents: Unregister\nExit") -> ("States Out"=w415:string)  [unwired: 12 in]
            n151 = call <vilib>:"Add State(s) to Queue__JKI_lib_State_Machine.vi"("State(s) in Front (\"\")"=w415, "State(s) in (\"\")"=w424) -> ("States Out"=w423:string)  [unwired: 13 in]
          }
          frame "---------- API ----------" {
            # "#CSM \"Category Seperator\"\nDo not put any code in this frame."
          }
          frame "API: Set Script" {
            # "#CSM API Example\nCopy/Rename this case for your own API"
            n152 = call "CSM - Revert Arguments-Safe String.vi"("Safe Argument String"=w432) -> ("Origin Argument String"=w433:string)  [unwired: 8 in]
            n153 = Bundle By Name(cluster=w436, "Script"=w433) -> (w434:T5)
            n154 = call <vilib>:"Add State(s) to Queue__JKI_lib_State_Machine.vi"("State(s) in (\"\")"=w430, "State(s) at Back (\"\")"="UI: Refresh Inputs" ("State(s) in Front (\"\")")) -> ("States Out"=w431:string)  [unwired: 13 in]
          }
          frame "---------- Action ----------" {
            # "#CSM \"Category Seperator\"\nDo not put any code in this frame."
            n155 = call <vilib>:"Add State(s) to Queue__JKI_lib_State_Machine.vi"("State(s) in (\"\")"=w442) -> ("States Out"=w441:string)  [unwired: 14 in]
          }
          frame "Action: Insert Last Resp Line" {
            n156 = Decimal String To Number(string=w456) -> (number=w453:i32)  [unwired: 2 in, 1 out]
            n157 = control-ref of="Script List"() -> (w455:refnum<vi>)
            n158 = call "Concatenate Submodule Name.vi"("Module Name"="CmdEditor", "Group Name"=w446) -> ("Submodule Name"=w444:string)  [unwired: 9 in]
            n159 = property class="LstBox (strict)"(reference=w455) -> (reference out=w451:refnum<vi>, "Item Names"=w454:string[])  [unwired: 1 in, 1 out]
            n160 = call "CSM - Send Message and Wait for Reply.vi"("Current Module (\"\" to Generate an ID)"=w446, "Target Module"=w444, "State"="API: Get Command") -> ("error out"=w447:errorcluster, "Response"=w449:string)  [unwired: 6 in, 1 out]
            n161 = call "CSM - Revert Arguments-Safe String.vi"("Safe Argument String"=w449) -> ("Origin Argument String"=w448:string)  [unwired: 8 in]
            n162 = Insert Into Array(array=w454, index=w453, new element=w448) -> (w452:string[])
            n163 = property class="LstBox (strict)"(reference=w451, "Item Names"=w452) -> ()  [unwired: 1 in, 2 out]
            n164 = call <vilib>:"Add State(s) to Queue__JKI_lib_State_Machine.vi"("State(s) in (\"\")"=w460, "State(s) at Back (\"\")"="Data: Redraw Scripts from UI" ("State(s) at Back (\"\")")) -> ("States Out"=w459:string)  [unwired: 13 in]
          }
          frame "Action: Replace Line" {
            n165 = Decimal String To Number(string=w473) -> (number=w470:i32)  [unwired: 2 in, 1 out]
            n166 = control-ref of="Script List"() -> (w472:refnum<vi>)
            n167 = call "Concatenate Submodule Name.vi"("Module Name"="CmdEditor", "Group Name"=w464) -> ("Submodule Name"=w462:string)  [unwired: 9 in]
            n168 = property class="LstBox (strict)"(reference=w472) -> (reference out=w468:refnum<vi>, "Item Names"=w471:string[])  [unwired: 1 in, 1 out]
            n169 = call "CSM - Send Message and Wait for Reply.vi"("Current Module (\"\" to Generate an ID)"=w464, "Target Module"=w462, "State"="API: Get Command") -> ("Response"=w465:string)  [unwired: 6 in, 2 out]
            n170 = call "CSM - Revert Arguments-Safe String.vi"("Safe Argument String"=w465) -> ("Origin Argument String"=w466:string)  [unwired: 8 in]
            n171 = Replace Array Subset(array=w471, new element=w466, index=w470) -> (w469:string[])
            n172 = property class="LstBox (strict)"(reference=w468, "Item Names"=w469) -> ()  [unwired: 1 in, 2 out]
            n173 = call <vilib>:"Add State(s) to Queue__JKI_lib_State_Machine.vi"("State(s) in (\"\")"=w478, "State(s) at Back (\"\")"="Data: Redraw Scripts from UI" ("State(s) at Back (\"\")")) -> ("States Out"=w477:string)  [unwired: 13 in]
          }
          frame "Action: Delete Line" {
            n174 = Decimal String To Number(string=w485) -> (number=w479:i32)  [unwired: 2 in, 1 out]
            n175 = control-ref of="Script List"() -> (w484:refnum<vi>)
            n176 = property class="LstBox (strict)"(reference=w484) -> (reference out=w481:refnum<vi>, "Item Names"=w483:string[])  [unwired: 1 in, 1 out]
            n177 = Delete From Array(array=w483, index=w479) -> (array with subset deleted=w482:string[])  [unwired: 1 in, 1 out]
            n178 = property class="LstBox (strict)"(reference=w481, "Item Names"=w482) -> ()  [unwired: 1 in, 2 out]
            n179 = call <vilib>:"Add State(s) to Queue__JKI_lib_State_Machine.vi"("State(s) in (\"\")"=w490, "State(s) at Back (\"\")"="Data: Redraw Scripts from UI" ("State(s) at Back (\"\")")) -> ("States Out"=w489:string)  [unwired: 13 in]
          }
        }
      }
      n180 = Unbundle By Name(w10) -> ("Script"=w9:string)
    }
    frame Error {
    }
  }
  "Error Out" <- w4
  "Script Out" <- w2
